vi "Toggle Component Display.vi"(8 "error in (no error)":errorcluster, 9 "Show":bool, 10 "Identifier":string, 11 "Main in":refnum<class "Main.lvclass">) -> (0 "error out":errorcluster, 3 "Main out":refnum<class "Main.lvclass">)   [LabVIEW 2023, in "Main.lvlib" / "Main.lvclass"]
uses:
  Library/Main.lvclass
  Library/Main.lvclass/Main.ctl
  builds/Framework/Engine.lvlibp/Managed Actor/Library/Managed Actor.lvclass
  builds/Framework/Panel Manager.lvlibp/Panel Actor/Panel Actor Messages/Hide Panel Msg/Hide Panel Msg.lvclass
  builds/Framework/Panel Manager.lvlibp/Panel Actor/Panel Actor Messages/Show Panel Msg/Show Panel Msg.lvclass
  builds/Main/Docking.lvlibp/Docking Messages/Adjust Splitter Msg/Adjust Splitter Msg.lvclass
  C:/Users/Public/Documents/Development/builds/Framework/Engine.lvlibp/Managed Actor/Library/Managed Actor.lvclass
  C:/Users/Public/Documents/Development/builds/Framework/Engine.lvlibp/Engine/Library/Engine.lvclass
  C:/Users/Public/Documents/Development/builds/Framework/Panel Manager.lvlibp/Library/Panel Actor.lvclass
  C:/Users/Public/Documents/Development/builds/Framework/Monitored Actor.lvlibp/Actor Monitor/Actor Monitor/Actor Monitor.lvclass
  C:/Users/Public/Documents/Development/builds/Framework/Actor Framework.lvlibp/1abvi3w/vi.lib/ActorFramework/Actor/Actor.lvclass
  C:/Users/Public/Documents/Development/Application/Main/Library/Main.lvclass
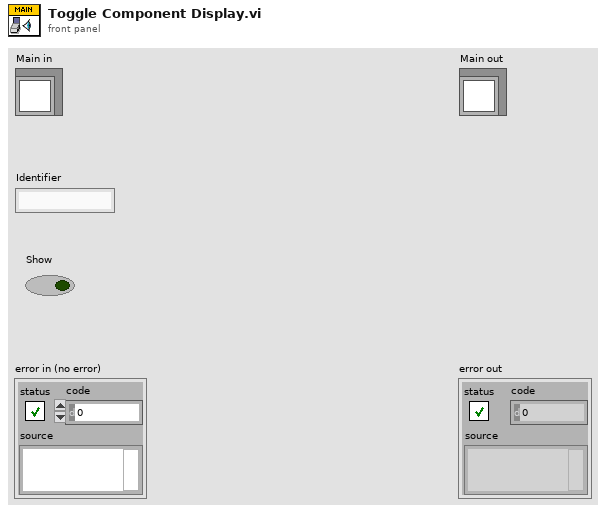
[diagram p1: front panel]
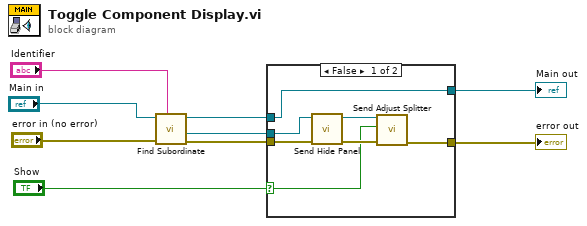
[diagram p0: block diagram]
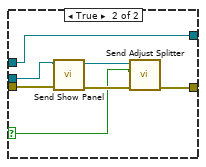
[diagram p2: hidden frame]
diagram:
  n1 = call "Find Subordinate.vi"("Identifier"="Identifier", "error in (no error)"="error in (no error)", "Managed Actor in"="Main in") -> ("error out"=w6:errorcluster, "Queue"=w4:refnum<class "Message Enqueuer.lvclass">, "Managed Actor out"=w5:refnum<class "Main.lvclass">)  [unwired: 4 in, 2 out]
  n2 = case shown="False" "Show" {
    selector: "Show" -> [w12 w18]
    tunnel: w6 -> [w16 w23]
    tunnel: w5 -> [w11 w21]
    tunnel: w4 -> [w15 w22]
    tunnel: [w11 w21] -> w3
    tunnel: [w10 w17] -> w1
    frame False {
      n3 = call "Send Hide Panel.vi"("error in (no error)"=w16, "Message Enqueuer in"=w15) -> ("error out"=w14:errorcluster, "Message Enqueuer out"=w13:refnum<class "Message Enqueuer.lvclass">)  [unwired: 8 in]
      n4 = call "Send Adjust Splitter.vi"("error in (no error)"=w14, "Show"=w12, "Message Enqueuer"=w13) -> ("error out"=w10:errorcluster)  [unwired: 7 in, 1 out]
    }
    frame True {
      n5 = call "Send Show Panel.vi"("Error In"=w23, "Message Enqueuer in"=w22) -> ("Error Out"=w20:errorcluster, "Message Enqueuer out"=w19:refnum<class "Message Enqueuer.lvclass">)  [unwired: 8 in]
      n6 = call "Send Adjust Splitter.vi"("error in (no error)"=w20, "Show"=w18, "Message Enqueuer"=w19) -> ("error out"=w17:errorcluster)  [unwired: 7 in, 1 out]
    }
  }
  "error out" <- w1
  "Main out" <- w3
